vi "Write ChannelInfo Changed Event 2.vi"(8 "error in (no error)":errorcluster, 10 "ChannelInfo Changed Event":refnum<user-event>, 11 "Channel in":refnum<class "Channel.lvclass">) -> (0 "error out":errorcluster, 3 "Channel out":refnum<class "Channel.lvclass">)   [LabVIEW 2015]
uses:
  Channel.lvclass
  ChannelInfo.lvclass
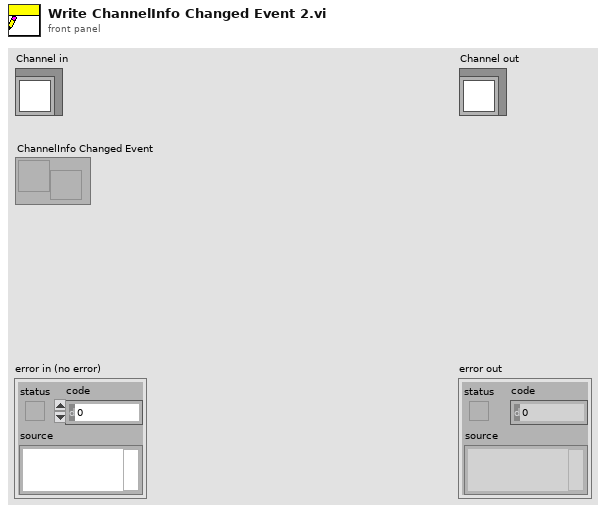
[diagram p1: front panel]
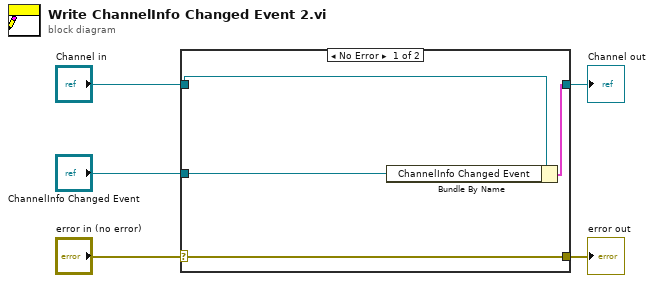
[diagram p0: block diagram]
diagram:
  n1 = case shown="No Error" "error in (no error)" {
    selector: "error in (no error)" -> [w9 w10]
    tunnel: [w9 w10] -> w4
    tunnel: [w7 w11] -> w2
    tunnel: "Channel in" -> [w8 w11]
    tunnel: "ChannelInfo Changed Event" -> [w6 _]
    frame No Error {
      n2 = Bundle By Name(cluster=w8, "ChannelInfo Changed Event"=w6) -> (w7:cluster{})
    }
    frame Error {
    }
  }
  "error out" <- w4
  "Channel out" <- w2
